vi "WLAN - TxMeasure - Test.vi"() -> ()   [LabVIEW 2012]
uses:
  TV/RW/Includes/WLAN - TV - RW - INC - Tx_IQModResult.ctl
  TV/RW/Includes/WLAN - NIStandardDefine.ctl
panel:
  in  "NeedMask?":bool=TRUE
  in  "pathloss":T1={"Pathloss Folder Path"=path "D:/4-Up WLAN Test System/Instrument Control/PL", "DUT Number"=0, "chain index"=1, "External Path Loss dB"=-10.0}
  in  "NIStandard":T2=enum."80211NMIMOOFDM"
  out "Margin VECTOR":dbl[](array[numeric])
  out "Mod Result":T3={"EVM"=0.0, "RMS POWER"=16.996999699969997, "FREQ ERR PPm"=0.0, "Clock ERR PPm"=0.0}
  out "error out 3":errorcluster={"status"=TRUE, "code"=-369023, "source"="niRFSA Fetch IQ (Complex Cluster 1Rec 1Chan).vi<ERR>Maximum time exceeded before the operation completed. "}
  out "error out 2":errorcluster
  out "SMM":dbl
  in  "stop":bool
  in  "RFSA":refnum<k15>="RIO0"
  in  "Center Frequency(Hz)":dbl=5790000000.0
  in  "Power Level(dBm)":dbl
  in  "Channel Bandwidth(Hz)":dbl=20000000.0
  out "error out":errorcluster
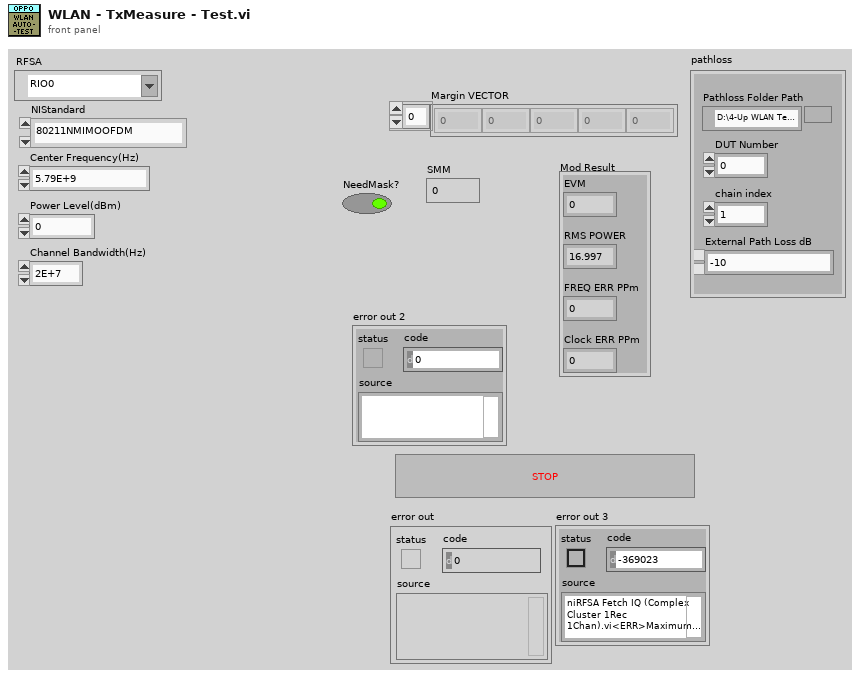
[diagram p1: front panel]
types:
  T1 = cluster{"Pathloss Folder Path":path, "DUT Number":i32, "chain index":i32, "External Path Loss dB":dbl}
  T2 = typedef "WLAN - NIStandardDefine.ctl" = enum32{"80211A/G/J/P(OFDM)", "80211B/G(DSSS)", "80211GDSSSOFDM", "80211NMIMOOFDM", "80211ACMIMOOFDM"}
  T3 = typedef "WLAN - TV - RW - INC - Tx_IQModResult.ctl" = cluster{"EVM":dbl, "RMS POWER":dbl, "FREQ ERR PPm":dbl, "Clock ERR PPm":dbl}
  T4 = typedef "wlanv1 Analysis Refnum.ctl" = refnum<k20>
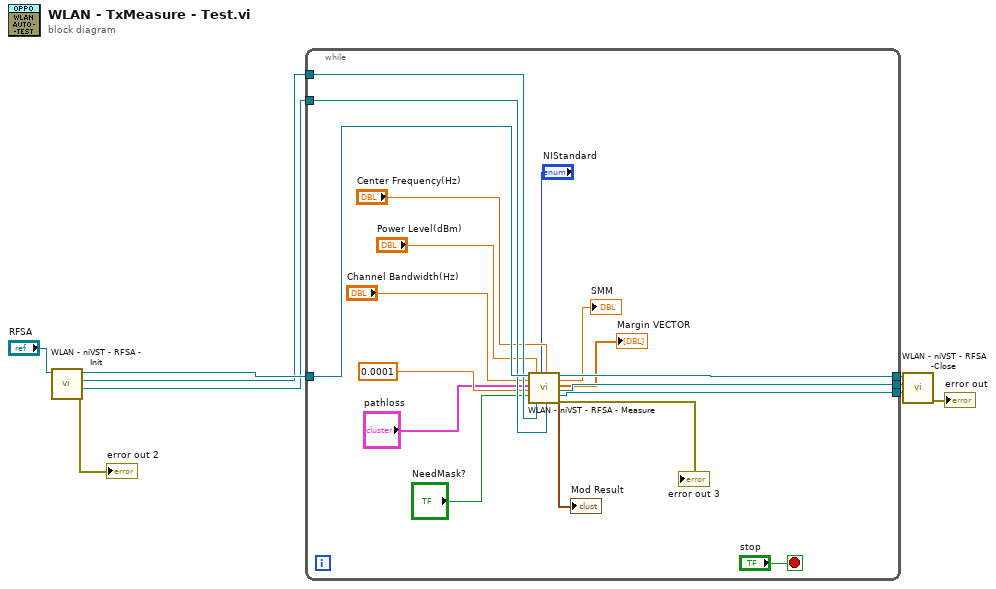
[diagram p0: block diagram]
diagram:
  n1 = call "WLAN - niVST - RFSA - Init.vi"("RFSA Handle In"="RFSA") -> ("error out"=→"error out 2":errorcluster, "IQ Meas Ref"=w5:T4, "Spectrum Meas Ref"=w4:T4, "RFSA Handle Out"=w6:refnum<k15>)  [unwired: 7 in]
  n2 = while {
    tunnel: [w27] -> w9
    tunnel: [w26] -> w8
    tunnel: [w25] -> w7
    tunnel: w6 -> [w24]
    tunnel: w5 -> [w23]
    tunnel: w4 -> [w22]
    stop <- "stop" stop-if-true
    n3 = call "WLAN - niVST - RFSA - Measure.vi"("RFSA Handle In"=w24, "Channel Bandwidth(Hz)"="Channel Bandwidth(Hz)", "pathloss"="pathloss", "Acquisition Length (s)"=0.0001, "NeedMask?"="NeedMask?", "Power Level(dBm)"="Power Level(dBm)", "Spectrum Meas Ref"=w22, "NIStandard"="NIStandard", "Center Frequency(Hz)"="Center Frequency(Hz)", "IQ Meas Ref"=w23) -> ("Mod Result"=→"Mod Result":T3, "RFSA Handle Out"=w27:refnum<k15>, "SMM"=→"SMM":dbl, "Margin VECTOR"=→"Margin VECTOR":dbl[], "Spectrum Meas Ref out"=w25:T4, "IQ Meas Ref out"=w26:T4, "error out"=→"error out 3":errorcluster)  [unwired: 3 in]
  }
  n4 = call "WLAN - niVST - RFSA -Close.vi"("IQ Meas Ref"=w8, "Spectrum Meas Ref"=w7, "RFSA Handle In"=w9) -> ("error out"=→"error out":errorcluster)  [unwired: 8 in]
